vi "RF Responsivity.vi"() -> ()   [LabVIEW 2018]
uses:
  <vilib>/express/express shared/transition.llb/Dynamic To Waveform Array.vi
  <vilib>/express/express signal manip/GetorSetDDTAttributes/Set DDT Attributes/SetT0.vi
  <vilib>/express/express shared/transition.llb/Waveform Array To Dynamic.vi
  <vilib>/express/express signal manip/GetorSetDDTAttributes/Set DDT Attributes/Set DDT Properties.xnode
panel:
  out "RF D":dbl
  out "RF C":dbl
  out "RF B":dbl
  out "RF A":dbl
  out "max value":dbl
  in  "Enable":bool=TRUE
  in  "Filename":path=path "C:/Users/physics-svc-fulda/Desktop/LabVIEW Data/DC A.lvm"
  in  "Signal Name":string
  out "Saving Data":bool
  out "Waveform Graph":dynamicdata(graph)
  out "RF Offset A":dbl format="%0.6f"
  out "RF Offset C":dbl format="%0.6f"
  out "RF Offset B":dbl format="%0.6f"
  out "RF Offset D":dbl format="%0.6f"
  in  "timeout (s)":dbl=10.0 format="%0.2f"
  in  "rate":dbl=1000.0
  in  "# of samples":i32=100
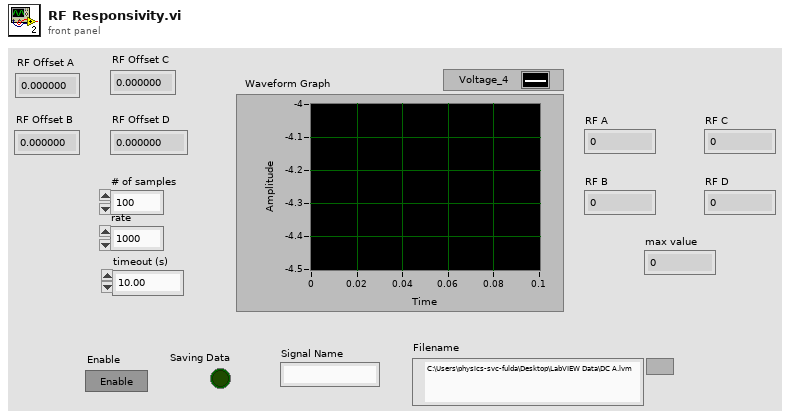
[diagram p1: front panel]
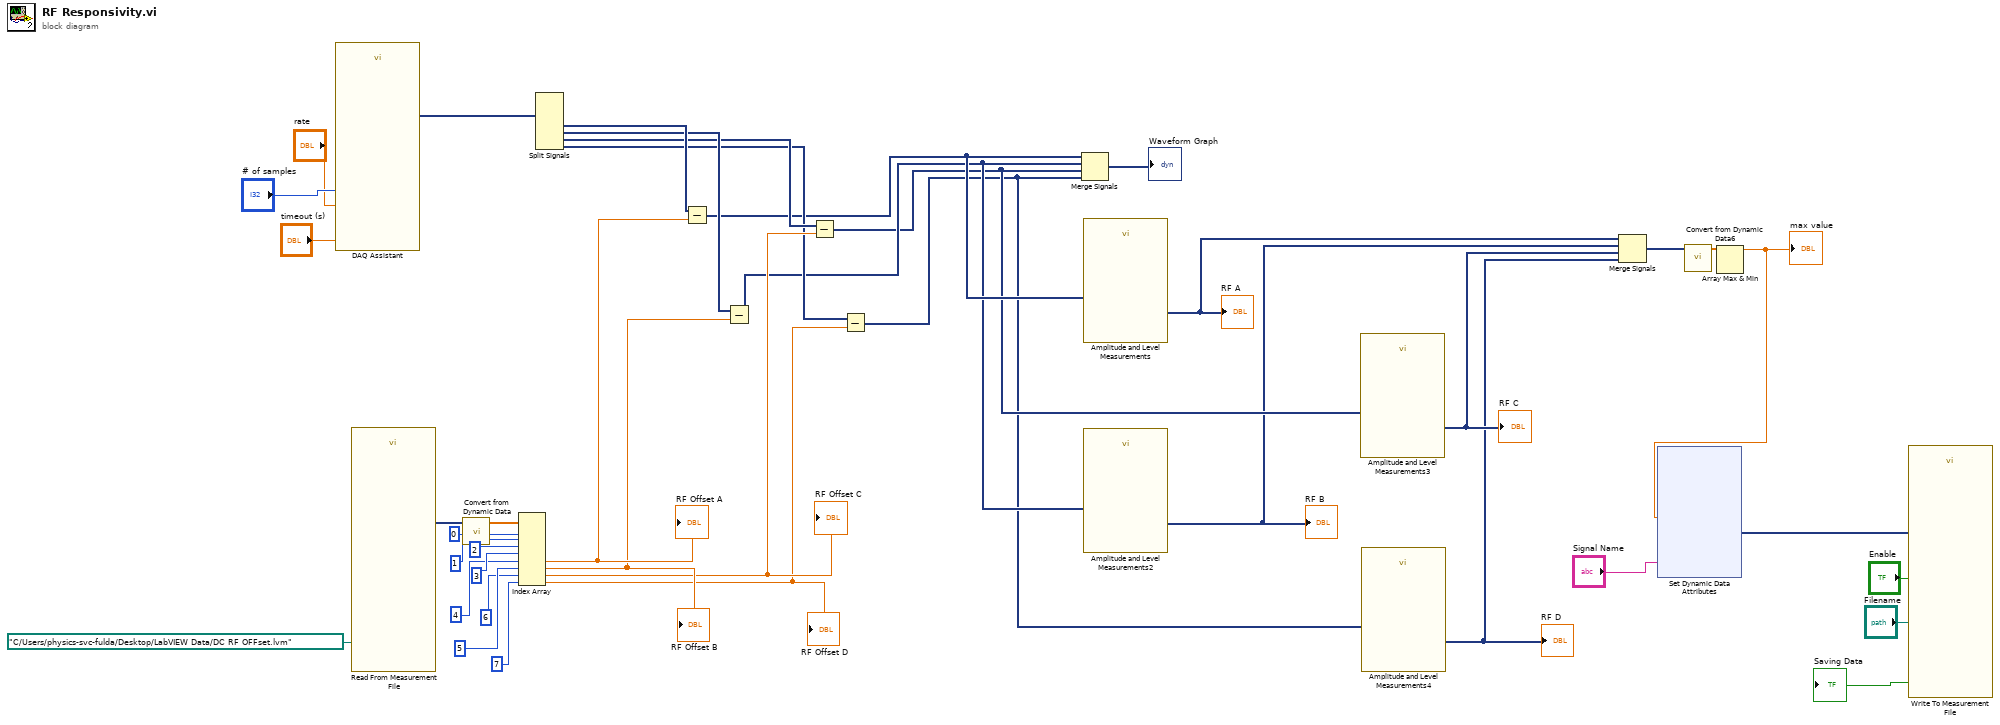
[diagram p0: block diagram]
diagram:
  n1 = call "DAQ Assistant"("rate"="rate", "number of samples"="# of samples", "timeout (s)"="timeout (s)") -> ("data"=w37:dynamicdata)  [unwired: 14 in, 2 out]
  n2 = call "Read From Measurement File"("Filename"=path "C:/Users/physics-svc-fulda/Desktop/LabVIEW Data/DC RF OFFset.lvm") -> ("Signals"=w34:dynamicdata)  [unwired: 5 in, 5 out]
  n3 = call "Convert from Dynamic Data"("Dynamic Data Type"=w34) -> ("Array"=w33:dbl[])  [unwired: 3 in]
  n4 = Index Array(array=w33, index #1=0 ("index"), index #2=1 ("index"), index #3=2 ("index"), index #4=3 ("index"), index #5=4 ("index"), index #6=5 ("index"), index #7=6 ("index"), index #8=7 ("index")) -> (element #5=w23:dbl, element #6=w22:dbl, element #7=w19:dbl, element #8=w17:dbl)  [unwired: 4 out]
  "RF Offset D" <- w17
  "RF Offset B" <- w22
  "RF Offset C" <- w19
  "RF Offset A" <- w23
  n5 = Split Signals(w37) -> (w24:dynamicdata, w21:dynamicdata, w20:dynamicdata, w18:dynamicdata)  [unwired: 8 in, 4 out]
  n6 = Subtract(x=w24, y=w23) -> (x-y=w8:dynamicdata)
  n7 = Subtract(x=w21, y=w22) -> (x-y=w6:dynamicdata)
  n8 = Subtract(x=w20, y=w19) -> (x-y=w5:dynamicdata)
  n9 = Subtract(x=w18, y=w17) -> (x-y=w4:dynamicdata)
  n10 = Merge Signals(w8, w6, w5, w4) -> (→"Waveform Graph":dynamicdata)
  n11 = call "Amplitude and Level Measurements"("Signals"=w8) -> ("Peak to Peak"=w7:dynamicdata)  [unwired: 13 in, 1 out]
  "RF A" <- w7
  n12 = call "Amplitude and Level Measurements2"("Signals"=w6) -> ("Peak to Peak"=w3:dynamicdata)  [unwired: 13 in, 1 out]
  "RF B" <- w3
  n13 = call "Amplitude and Level Measurements3"("Signals"=w5) -> ("Peak to Peak"=w2:dynamicdata)  [unwired: 13 in, 1 out]
  "RF C" <- w2
  n14 = call "Amplitude and Level Measurements4"("Signals"=w4) -> ("Peak to Peak"=w1:dynamicdata)  [unwired: 13 in, 1 out]
  "RF D" <- w1
  n15 = Merge Signals(w7, w3, w2, w1) -> (w11:dynamicdata)
  n16 = call "Convert from Dynamic Data6"("Dynamic Data Type"=w11) -> ("Array"=w10:dbl[])  [unwired: 3 in]
  n17 = Array Max & Min(array=w10) -> (max value=w9:dbl)  [unwired: 3 out]
  "max value" <- w9
  n18 = xnode "Set Dynamic Data Attributes"("Signals In"=w9, "Signal Name"="Signal Name") -> ("Signals Out"=w15:dynamicdata)  [unwired: 2 in, 1 out]
  n19 = call "Write To Measurement File"("Signals"=w15, "Enable"="Enable", "Filename"="Filename") -> ("Saving Data"=→"Saving Data":bool)  [unwired: 14 in, 2 out]
